vi "rmx13_rev2 - Copy.vi"() -> ()   [LabVIEW 2012]
uses:
  <vilib>/LabVIEW Interface for Arduino/Type Defs/Connection Type.ctl
  <vilib>/LabVIEW Interface for Arduino/Type Defs/Board Type.ctl
  <vilib>/Utility/inputDevices.llb/closeKeyboard.vi
  <vilib>/Utility/inputDevices.llb/keyboardAcquire.vi
  <vilib>/LabVIEW Interface for Arduino/LabVIEW Interface for Arduino.lvlib
panel:
  out "String 2":string
  in  "Tab Control 2":enum32{"Settings", "Page 2"}(tab)
  in  "VISA resource name":refnum<visa-resource-name>
  in  "Baud Rate":u32
  in  "Connection Type":T1
  in  "Board Type":T2
  out "Error Out":errorcluster
  in  "Tab Control":enum32{"Front Panel"}(tab)
  out "xdown":bool
  out "xup":bool
  in  "Boolean 2":bool
  out "excavator direction":string="a"
  out "bot direction":string="a"
  out "excavator state":string="a"
  out "hopper state":string="a"
  out "bytes written":i32
  out "tx'd string":string
  out "error out":errorcluster
  out "Total Elapsed Time  (HH:MM:SS)":dbl format="%<%H:%M:%S%2u>t"
  in  "Boolean":bool
  out "hup":bool
  out "hdown":bool
  out "xfwd":bool
  out "xback":bool
  out "right":bool
  out "left":bool
  out "down":bool
  out "up":bool
  # "Excavator State"
  # "Elapsed Time"
  # "Dump Position"
  # "Excavator Direction"
  # "Start/Stop"
  # "Bot Direction"
  # "Hopper State"
  # "Error Control"
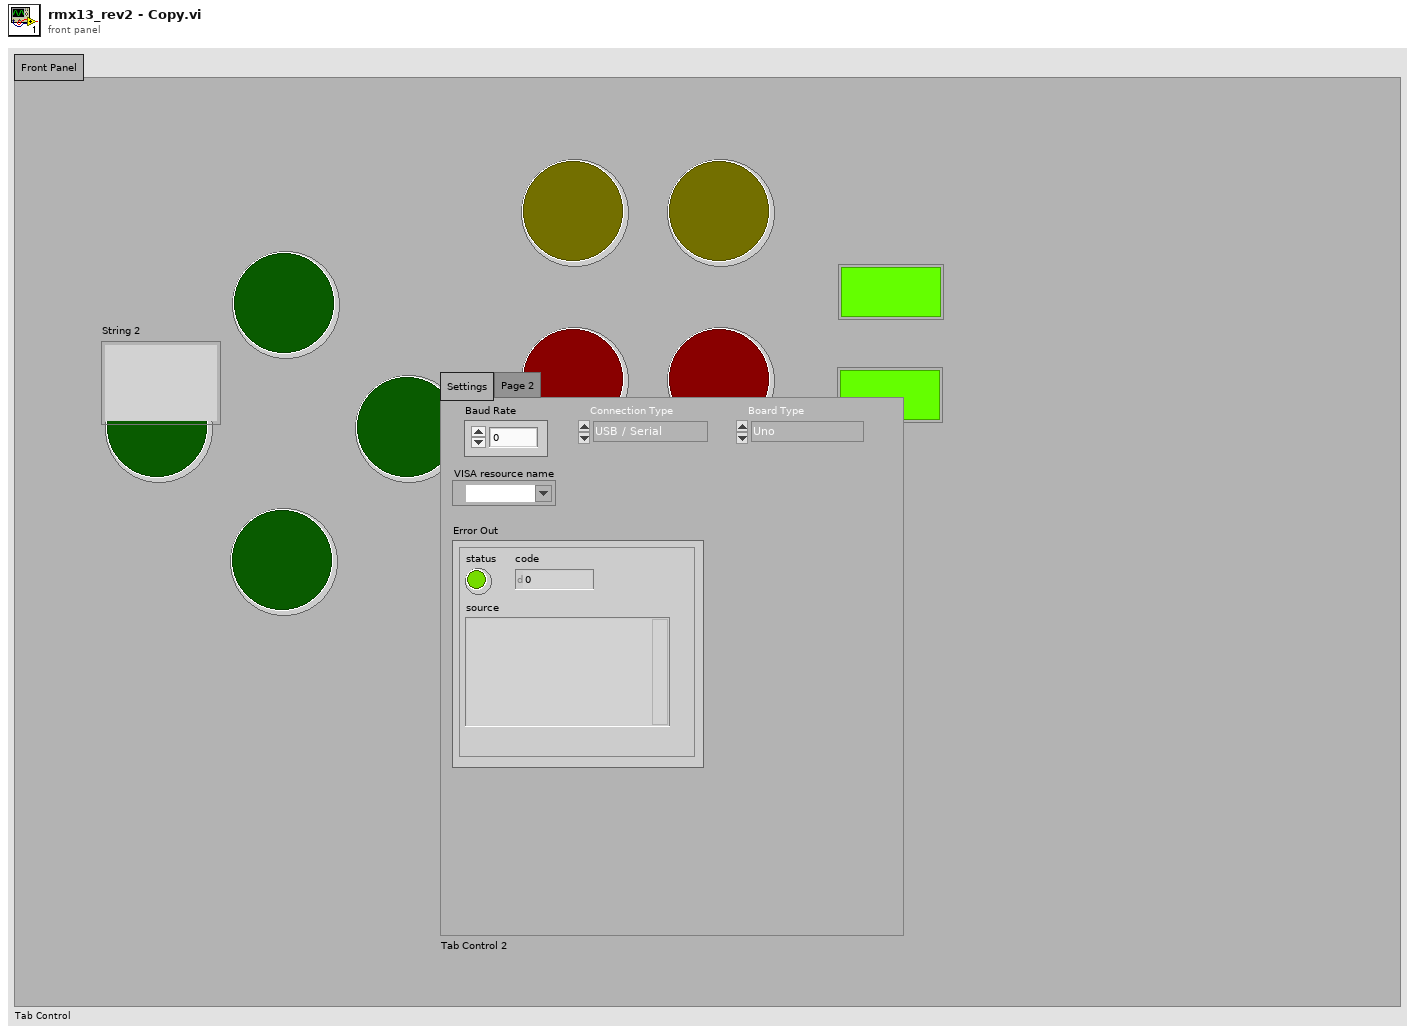
[diagram p1: front panel]
types:
  T1 = typedef "LabVIEW Interface for Arduino.lvlib/Connection Type.ctl" = enum8{"USB / Serial", "XBEE", "BlueSmirf (Bluetooth)"}
  T2 = typedef "LabVIEW Interface for Arduino.lvlib/Board Type.ctl" = enum16{"Uno", "Dimuelanove w/Atmega 328", "Mega 2560"}
  T3 = typedef "LabVIEW Interface for Arduino.lvlib/Arduino Resource.ctl" = cluster{"VISA resource":refnum<visa-resource-name>, "Board Type":T2, "Connection Type":enum8{"USB / Serial"}, "Bytes Per Packet (15)":u8}
  T4 = enum16{"0", "1", "2", "3", "4", "5", "6", "7", "8", "9", "A", "B", "C", "D", "E", "F", "G", "H", "I", "J", "K", "L", "M", "N", "O", "P", "Q", "R", "S", "T", "U", "V", "W", "X", "Y", "Z", "F1", "F2", "F3", "F4", "F5", "F6", "F7", "F8", "F9", "F10", "F11", "F12", "F13", "F14", "F15", "ADD", "BACK", "BACKSLASH", "CAPITAL", "COMMA", "DECIMAL", "DELETE", "DIVIDE", "DOWN", "END", "EQUALS", "ESCAPE", "GRAVE (`)", "HOME", "INSERT", "LBRACKET", "LCONTROL", "LEFT", "L ALT", "LSHIFT", "LWIN", "MINUS", "MULTIPLY", "NEXT", "NUMLOCK", "NUMPAD_0", "NUMPAD_1", "NUMPAD_2", "NUMPAD_3", "NUMPAD_4", "NUMPAD_5", "NUMPAD_6", "NUMPAD_7", "NUMPAD_8", "NUMPAD_9", "PAUSE", "PERIOD", "PRIOR (PG UP)", "RBRACKET", "RCONTROL", "RETURN", "RIGHT", "R ALT", "RSHIFT", "RWIN", "SCROLL", "SEMICOLON", "SLASH", "SPACE", "SUBTRACT", "TAB", "UP", "ENTER (num pad)", "' (quote)"}[]
  T5 = cluster{"up":bool, "down":bool, "left":bool, "right":bool, "xup":bool, "xdown":bool, "hup":bool, "hdown":bool, "xfwd":bool, "xback":bool}
  T6 = cluster{"bot_dir":string, "x-state":string, "h-state":string, "x-dir":string}
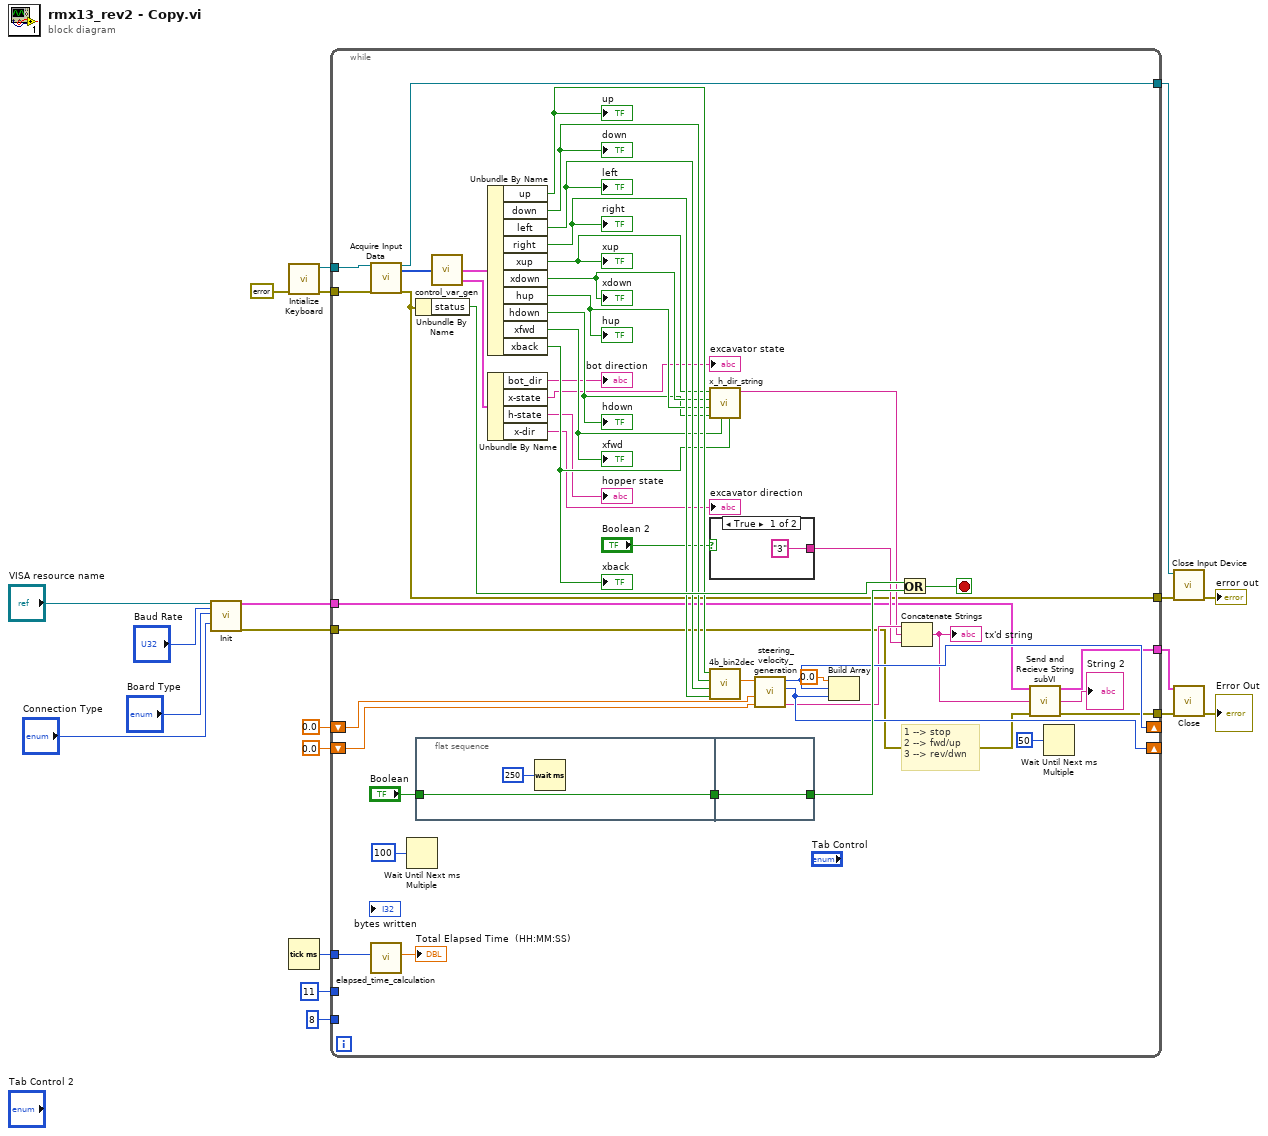
[diagram p0: block diagram]
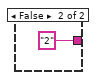
[diagram p2: hidden frame]
diagram:
  n1 = call <vilib>:"Init.vi"("VISA resource"="VISA resource name", "Baud Rate (115200)"="Baud Rate", "Board Type (Uno)"="Board Type", "Connection Type (USB/Serial)"="Connection Type") -> ("Arduino Resource"=w6:T3, "error out"=w5:errorcluster)  [unwired: 14 in]
  n2 = call <vilib>:"Intialize Keyboard.vi"("error in (no error)"=errorcluster {"status"=FALSE, "code"=0, "source"=""} ("error in")) -> ("error out"=w19:errorcluster, "device ID"=w20:refnum<k1>)  [unwired: 9 in]
  n3 = Tick Count (ms)() -> (millisecond timer value=w16:u32)
  n4 = while {
    tunnel: w20 -> [w66]
    tunnel: w19 -> [w65]
    tunnel: [w62] -> w18
    tunnel: [w28] -> w17
    tunnel: w16 -> [w48]
    shift-right: [w50] -> _
    shift-left: 0.0 -> [w52]
    shift-right: [w49] -> _
    shift-left: 0.0 -> [w51]
    tunnel: w6 -> [w24]
    tunnel: w5 -> [w23]
    tunnel: [w22] -> w4
    tunnel: [w21] -> w3
    tunnel: 11 -> [_]
    tunnel: 8 -> [_]
    stop <- w54 stop-if-true
    # "1 --> stop\n2 --> fwd/up\n3 --> rev/dwn"
    n5 = call-poly <vilib>:"Acquire Input Data.vi"("device ID"=w66, "error in (no error)"=w65) -> ("device ID"=w62:refnum<k1>, "keys pressed"=w61:T4, "error out"=w28:errorcluster)  [unwired: 15 in]
    n6 = call "elapsed_time_calculation.vi"("initial time"=w48) -> ("elapsed time"=→"Total Elapsed Time  (HH:MM:SS)":dbl)  [unwired: 10 in]
    n7 = Wait Until Next ms Multiple(millisecond multiple=u32 100) -> ()  [unwired: 1 out]
    n8 = Unbundle By Name(w28) -> ("status"=w56:bool)
    n9 = flat-sequence {
      tunnel: "Boolean" -> [w69]
      tunnel: [w69] -> w64
      tunnel: [w71] -> w55
      tunnel: w64 -> [w71]
      frame #0 {
        n10 = Wait (ms)(milliseconds to wait=u32 250) -> ()  [unwired: 1 out]
      }
      frame #1 {
      }
    }
    n11 = call "control_var_gen.vi"("keys pressed"=w61) -> ("out_panel"=w60:T5, "out_error"=w59:T6)  [unwired: 5 in]
    n12 = Unbundle By Name(w60) -> ("up"=w46:bool, "down"=w45:bool, "left"=w44:bool, "right"=w43:bool, "xup"=w42:bool, "xdown"=w41:bool, "hup"=w40:bool, "hdown"=w39:bool, "xfwd"=w38:bool, "xback"=w37:bool)
    "up" <- w46
    "down" <- w45
    "left" <- w44
    "right" <- w43
    "xup" <- w42
    "xdown" <- w41
    "hup" <- w40
    "hdown" <- w39
    "xfwd" <- w38
    "xback" <- w37
    n13 = Unbundle By Name(w59) -> ("bot_dir"=→"bot direction":string, "x-state"=→"excavator state":string, "h-state"=→"hopper state":string, "x-dir"=→"excavator direction":string)
    n14 = call "x_h_dir_string.vi"("xback"=w37, "xfwd"=w38, "hdown"=w39, "hup"=w40, "xdown"=w41, "xup"=w42) -> ("x_h_dir"=w35:string)  [unwired: 5 in]
    n15 = case shown="True" "Boolean 2" {
      tunnel: ["3" "2"] -> w33
      frame True {
      }
      frame False {
      }
    }
    n16 = call "4b_bin2dec.vi"("Right"=w43, "Left"=w44, "Down"=w45, "Up"=w46) -> ("Out"=w53:dbl)  [unwired: 7 in]
    n17 = call "steering_velocity_generation.vi"("angular velocity"=w51, "forward velocity"=w52, "bool-to-dec value"=w53) -> ("motor_control_sig"=w36:string, "angular velocity 2"=w49:i32, "forward velocity 2"=w50:i32)  [unwired: 6 in]
    n18 = Build Array(0.0 ("element"), w50, w49) -> ()  [unwired: 1 out]
    n19 = Or(x=w56, y=w55) -> (x .or. y?=w54:bool)
    n20 = Concatenate Strings(w36, w35, w33) -> (w25:string)
    "tx'd string" <- w25
    n21 = call "Send and Recieve String subVI.vi"("Arduino Resource"=w24, "String"=w25, "error in"=w23) -> ("Arduino Resource 2"=w22:T3, "String Output"=→"String 2":string, "error out"=w21:errorcluster)  [unwired: 10 in]
    n22 = Wait Until Next ms Multiple(millisecond multiple=u32 50) -> ()  [unwired: 1 out]
  }
  n23 = call-poly <vilib>:"Close Input Device.vi"("error in (no error)"=w17, "device ID"=w18) -> ("error out"=→"error out":errorcluster)  [unwired: 8 in]
  n24 = call <vilib>:"Close.vi"("Arduino Resource"=w4, "error in"=w3) -> ("error out"=→"Error Out":errorcluster)  [unwired: 13 in]
